vi "InTake Problem Fix.vi"(1 "InTake Global Data Modified":T1, 2 "InTake Global Data Original":T1) -> (0 "InTake Global Data New":T1)   [LabVIEW 2013]
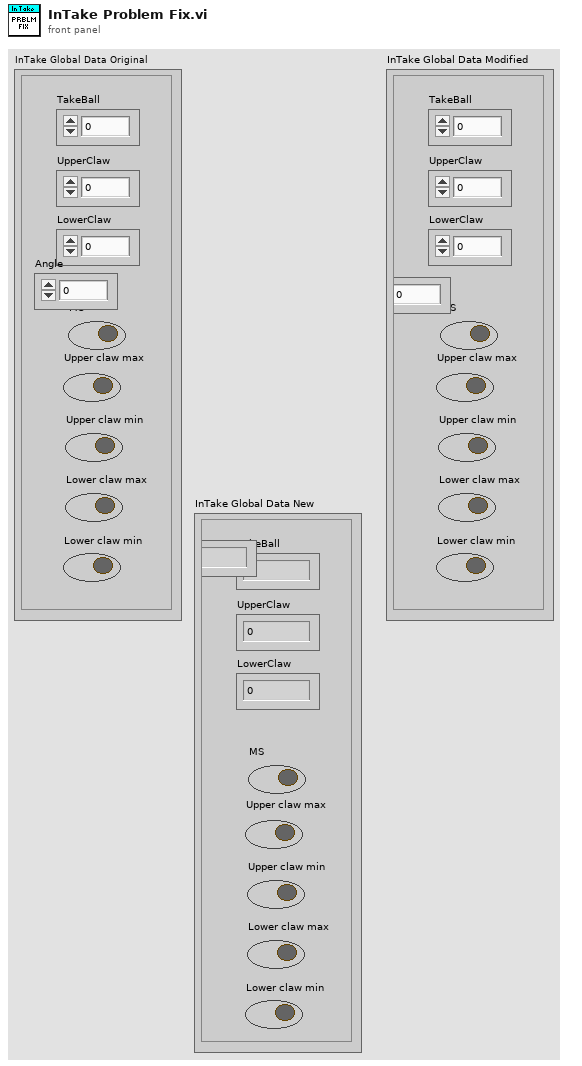
[diagram p1: front panel]
types:
  T1 = cluster{"TakeBall":dbl, "UpperClaw":dbl, "LowerClaw":dbl, "MS":bool, "Upper claw max":bool, "Lower claw max":bool, "Upper claw min":bool, "Lower claw min":bool, "Angle":dbl}
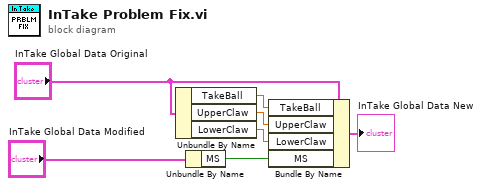
[diagram p0: block diagram]
diagram:
  n1 = Unbundle By Name("InTake Global Data Original") -> ("TakeBall"=w6:dbl, "UpperClaw"=w5:dbl, "LowerClaw"=w4:dbl)
  n2 = Unbundle By Name("InTake Global Data Modified") -> ("MS"=w3:bool)
  n3 = Bundle By Name(cluster="InTake Global Data Original", "TakeBall"=w6, "UpperClaw"=w5, "LowerClaw"=w4, "MS"=w3) -> (→"InTake Global Data New":T1)
